vi "Power & Time.vi"() -> ()   [LabVIEW 2017]
uses:
  Control 1.ctl
  <vilib>/Instr/_visa.llb/VISA Flush IO Buffer Mask.ctl
  <vilib>/Instr/_visa.llb/VISA Configure Serial Port (Instr).vi
panel:
  in  "?":bool
  out "CLOSE 5":T1 format="%#.8g"
  out "CLOSE 4":T1 format="%#.8g"
  out "CLOSE 3":T1 format="%#.8g"
  out "CLOSE 2":T1 format="%#.8g"
  out "CLOSE 1":T1 format="%#.8g"
  out "OPEN 5":T1 format="%#.8g"
  out "OPEN 4":T1 format="%#.8g"
  out "OPEN 3":T1 format="%#.8g"
  out "OPEN 2":T1 format="%#.8g"
  out "OPEN 1":T1 format="%#.8g"
  in  "TEST                     CALIBRATION":bool
  out "Total Average :":T1 format="%#.8g"
  out "CAL/FLT":bool
  out "TEST Open/Close":bool
  out "?":dbl(graph)
  out "Meter":ext(knob) scale=0.008..8.0
  in  "Start":bool
  in  "USB Port":refnum<visa-resource-name>
  in  "Baud rate (115200)":u32=9600
  in  "Parity (0:none)":enum16{"None", "Odd", "Even", "Mark", "Space"}(ring)
  in  "Data bits (8)":u16=8 min=5 max=8 step=1
  in  "S.B (10:1 bit)":u16(ring)=10 items=["1.0"=10, "1.5"=15, "2.0"=20]
  in  "FC   (None)":u16(ring) items=["None", "XON/XOFF", "RTS/CTS", "XON/XOFF & RTS/CTS", "DTR/DSR", "XON/XOFF & DTR/DSR"]
  # "Copyright © 2020 Tarfand inc                                                                                                                                                                                                                                                                       All rights reserved by : P.M"
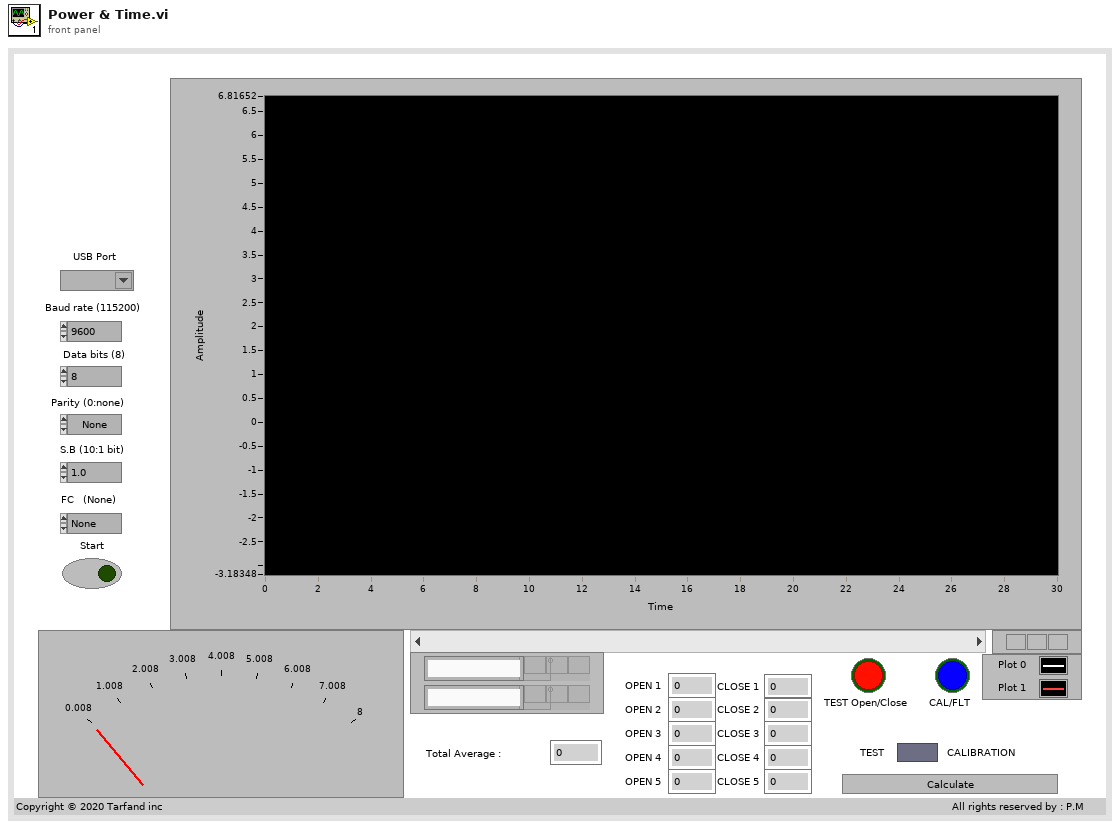
[diagram p1: front panel]
types:
  T1 = typedef "Control 1.ctl" = dbl
  T2 = typedef "VISA Flush IO Buffer Mask.ctl" = u16
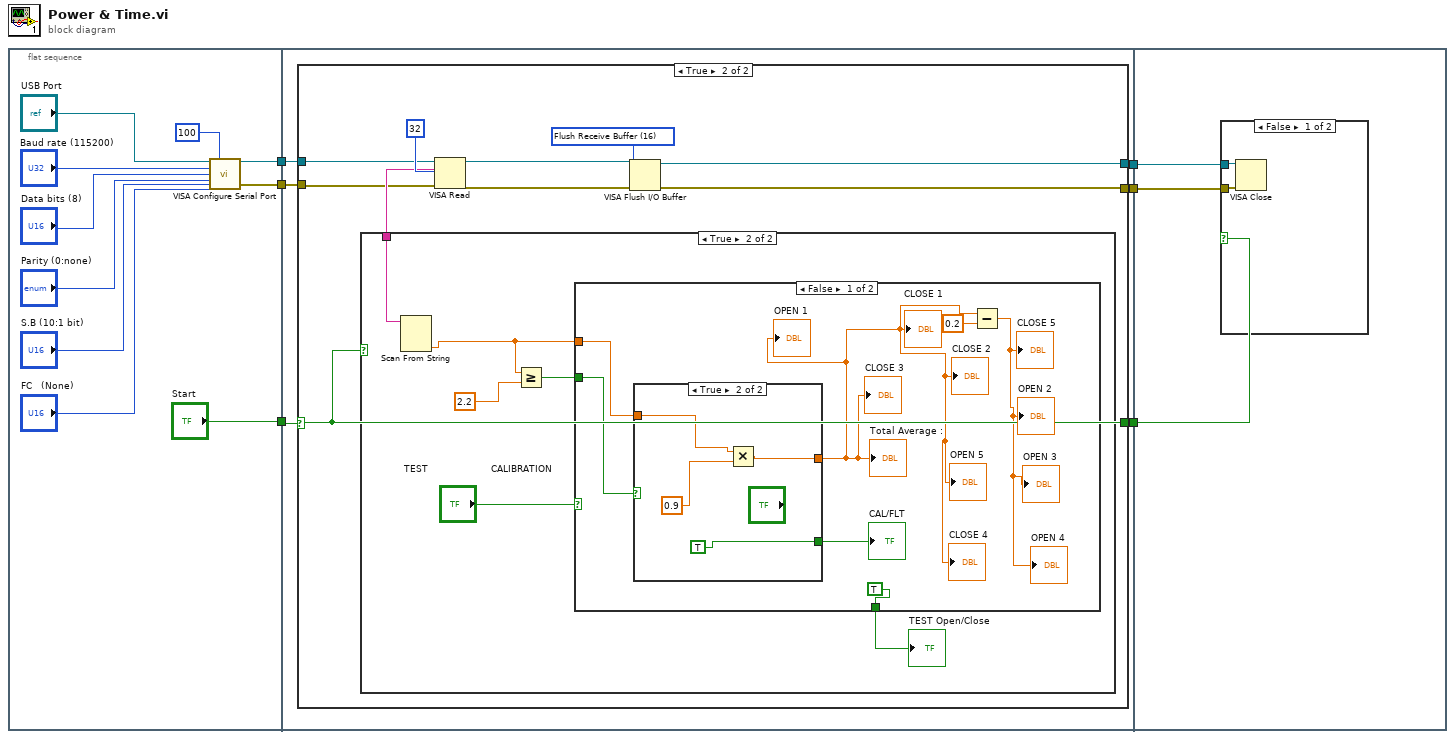
[diagram p0: block diagram]
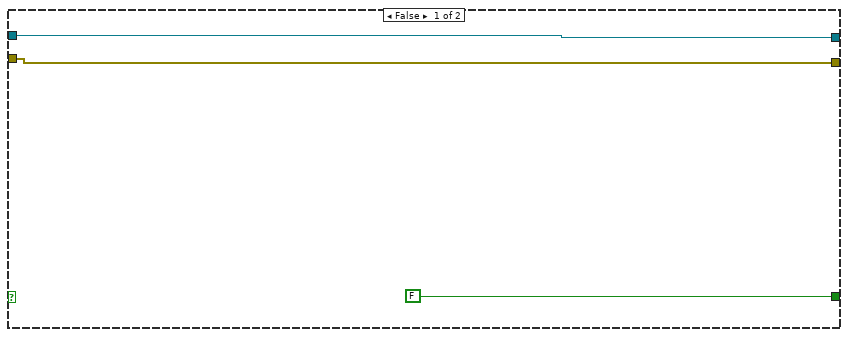
[diagram p2: hidden frame]
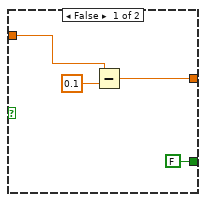
[diagram p4: hidden frame]
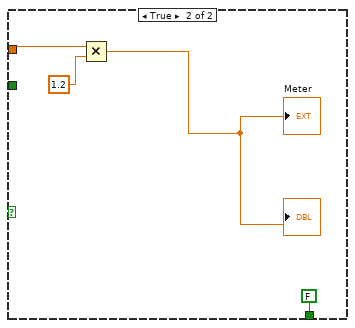
[diagram p5: hidden frame]
diagram:
  n1 = flat-sequence {
    tunnel: [w9] -> w6
    tunnel: [w10] -> w5
    tunnel: ["Start"] -> w2
    tunnel: w6 -> [w22]
    tunnel: w5 -> [w21]
    tunnel: [w20] -> w4
    tunnel: [w19] -> w3
    tunnel: w2 -> [w17]
    tunnel: [w18] -> w1
    tunnel: w4 -> [w63]
    tunnel: w3 -> [w62]
    tunnel: w1 -> [w61]
    frame #0 {
      n2 = call-poly "VISA Configure Serial Port"("VISA resource name"="USB Port", "timeout (10sec)"=u32 100, "baud rate (9600)"="Baud rate (115200)", "data bits (8)"="Data bits (8)", "parity (0:none)"="Parity (0:none)", "stop bits (10: 1 bit)"="S.B (10:1 bit)", "flow control (0:none)"="FC   (None)") -> ("VISA resource name out"=w9:refnum<visa-resource-name>, "error out"=w10:errorcluster)  [unwired: 7 in]
    }
    frame #1 {
      n3 = case shown="True" w17 {
        selector: w17 -> [_ w29]
        tunnel: w22 -> [w25 w31]
        tunnel: w21 -> [w24 w26]
        tunnel: [w25 w30] -> w20
        tunnel: [w24 w28] -> w19
        tunnel: [FALSE w29] -> w18
        frame False {
        }
        frame True {
          w35 = T2 16 items=["Flush Receive Buffer"=16, "Write Transmit Buffer to Device"=32, "Flush Receive Buffer (No I/O)"=64, "Flush Transmit Buffer"=128] ("Mask")
          n4 = VISA Read(VISA resource name=w31, byte count=u32 32, error in (no error)=w26) -> (VISA resource name out=w34:refnum<visa-resource-name>, read buffer=w32:string, error out=w27:errorcluster)  [unwired: 1 out]
          n5 = case shown="True" w29 {
            tunnel: w32 -> [_ w41]
            frame False {
            }
            frame True {
              n6 = Scan From String(input string=w41) -> (output 1=w37:dbl)  [unwired: 4 in, 3 out]
              n7 = Greater Or Equal?(x=w37, y=2.2) -> (x >= y?=w38:bool)
              n8 = case shown="False" "TEST                     CALIBRATION" {
                tunnel: w37 -> [w48 w60]
                tunnel: w38 -> [w47 _]
                tunnel: [TRUE ("Boolean") FALSE ("Boolean")] -> w36
                frame False {
                  n9 = case shown="True" w47 {
                    tunnel: w48 -> [w51 w54]
                    tunnel: [w52 w55] -> w43
                    tunnel: [FALSE ("CAL/FLT") TRUE ("CAL/FLT")] -> w46
                    frame False {
                      n10 = Subtract(x=w51, y=0.1) -> (x-y=w52:dbl)
                    }
                    frame True {
                      n11 = Multiply(x=w54, y=0.9) -> (x*y=w55:dbl)
                    }
                  }
                  "Total Average :" <- w43
                  "CAL/FLT" <- w46
                  "CLOSE 1" <- w43
                  "CLOSE 2" <- w43
                  "OPEN 5" <- w43
                  "CLOSE 4" <- w43
                  "CLOSE 3" <- w43
                  "OPEN 1" <- w43
                  n12 = Subtract(x=w43, y=0.2) -> (x-y=→"OPEN 2" →"OPEN 3" →"OPEN 4" →"CLOSE 5":dbl)
                }
                frame True {
                  n13 = Multiply(x=w60, y=1.2) -> (x*y=→"Meter" →"?":dbl)
                }
              }
              "TEST Open/Close" <- w36
            }
          }
          n14 = VISA Flush I/O Buffer(VISA resource name=w34, mask (16)=w35, error in (no error)=w27) -> (VISA resource name out=w30:refnum<visa-resource-name>, error out=w28:errorcluster)
        }
      }
    }
    frame #2 {
      n15 = case shown="False" w61 {
        tunnel: w63 -> [w64 _]
        tunnel: w62 -> [w65 _]
        frame False {
          n16 = VISA Close(VISA resource name=w64, error in (no error)=w65) -> ()  [unwired: 1 out]
        }
        frame True {
        }
      }
    }
  }
